vi "Main.vi"() -> ()   [LabVIEW 2017]
uses:
  <vilib>/Platform/TimedLoop/XDataNode/timing_clust.ctl
  <vilib>/Platform/TimedLoop/XDataNode/nitl_modes.ctl
  <vilib>/Platform/TimedLoop/XDataNode/wakeup.ctl
  <instrlib>/_niInstr/Instruction Framework/v1/FPGA/Helper Classes/Single Address Space Collection/Single Address Space Collection.lvclass
  C:/Program Files (x86)/National Instruments/LabVIEW 2017/instr.lib/_niInstr/Instruction Framework/v1/FPGA/Interfaces/Address Space Collection/Address Space Collection.lvclass
  <instrlib>/_niInstr/FIFO Register Bus/v1/FPGA/niInstr FIFO Register Bus v1 FPGA.lvclass
  C:/Program Files (x86)/National Instruments/LabVIEW 2017/instr.lib/_niInstr/Instruction Framework/v1/FPGA/Interfaces/Instruction Producer/Instruction Producer.lvclass
  <vilib>/rvi/Emulation/niFpgaGetClockAttributes.vi
  <vilib>/rvi/Emulation/niFpgaSctlEmulationGetInTimedLoop.vi
  <vilib>/rvi/Emulation/niFpgaEmulationReportErrorSimple.vi
  <vilib>/rvi/eio/common/nirviEmuTemplateMethod_errors.vi
  <vilib>/rvi/Emulation/niFpgaCriticalErrorInLSC.vi
  <vilib>/eio/EIONode/EIONode.xnode
  <vilib>/Platform/TimedLoop/XDataNode/XDataNode.xnode
  <instrlib>/_niInstr/Instruction Framework/v1/FPGA/Top Level Bus/Register Configuration/Register Configuration.lvclass
  Oscillator/Oscillator.lvclass
  <vilib>/Platform/TimedLoop/XDataNode/XDNodeRunTimeDep.lvlib
panel:
  in  "Enable?":bool
  out "Loop":i32
  in  "Signal Offset":i16
  in  "Signal Amplitude (x 2^15)":u16
  in  "Phase Shift":u32
  in  "Accumulator Increment":u32
  in  "Reset Accumulator":bool
  in  "Count(Ticks)":u32
  out "Actual Rate (ticks)":u32
  out "fifo reg bus data 0":u64
  out "fifo reg bus status 0":u32
  in  "fifo reg bus ctrl 0":u32
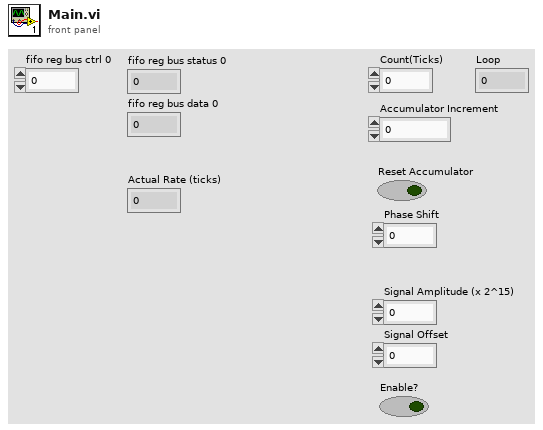
[diagram p1: front panel]
types:
  T1 = typedef "XDNodeRunTimeDep.lvlib/timing_clust.ctl" = cluster{"Expected End [f-1]":u64, "Actual End [f-1]":u64, "Finished Late? [f-1]":bool, "Expected End [i-1]":u64, "Actual End [i-1]":u64, "Finished Late? [i-1]":bool, "Expected Start [i]":u64, "Actual Start [i]":u64, "Expected Start [f]":u64, "Actual Start [f]":u64, "Source Name":string, "Structure Name":string, "Period":i64, "Deadline":i64, "Offset":i64, "Start":i64, "Priority":i32, "Timeout":i32, "Mode":T2, "Wakeup Reason":T3, "Error":errorcluster, "Source Type":string, "Secondary Source Type":string, "Global End Time":u64, "Global Start Time":u64, "Frame Duration":u64, "Iteration Duration":u64, "Assigned CPU":i32, "I/O Scan Engine Mode":u32}
  T2 = typedef "XDNodeRunTimeDep.lvlib/nitl_modes.ctl" = enum32{"No Change", "Process missed periods, maintain original phase", "Discard missed periods, maintain original phase", "Process missed periods, ignore original phase", "Discard missed periods, ignore original phase"}
  T3 = typedef "XDNodeRunTimeDep.lvlib/wakeup.ctl" = enum32{"Normal", "Aborted", "Asynchronous wakeup", "Timing source error", "Timed loop error", "Timeout"}
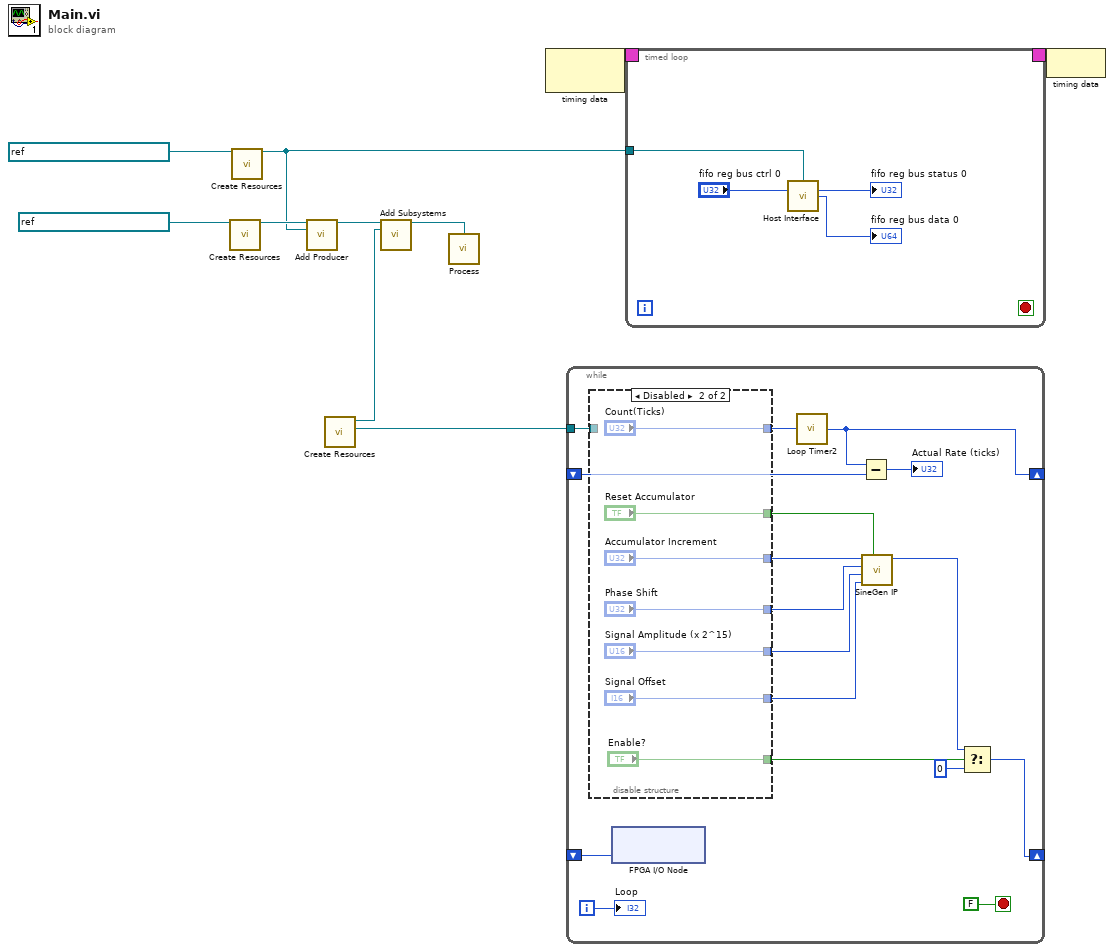
[diagram p0: block diagram]
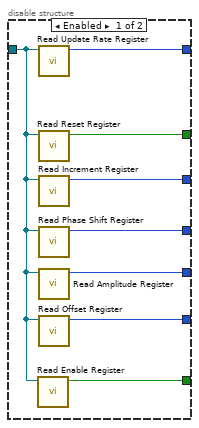
[diagram p2: hidden frame]
diagram:
  n1 = call <instrlib>:"Create Resources.vi"("register clock"=refnum<k21> "40 MHz Onboard Clock") -> ("register configuration"=w7:refnum<class "Register Configuration.lvclass">)  [unwired: 14 in]
  n2 = call <instrlib>:"Create Resources.vi"("instruction fifo"=refnum<k21> "reg.host instruction fifo 0") -> ("fifo register bus"=w5:refnum<class "niInstr FIFO Register Bus v1 FPGA.lvclass">)  [unwired: 14 in]
  n3 = call <instrlib>:"Add Producer.vi"("register configuration in"=w7, "instruction producer"=w5) -> ("register configuration out"=w4:refnum<class "Register Configuration.lvclass">)  [unwired: 13 in]
  n4 = call <instrlib>:"Create Resources.vi"() -> ("Oscillator Address Space out"=w1:refnum<class "Oscillator.lvclass">, "Subsystem out"=w3:refnum<class "Single Address Space Collection.lvclass">)  [unwired: 10 in]
  n5 = call <instrlib>:"Add Subsystems.vi"("register configuration in"=w4, "subsystems"=w3) -> ("register configuration out"=w2:refnum<class "Register Configuration.lvclass">)  [unwired: 13 in]
  n6 = call <instrlib>:"Process.vi"("register configuration"=w2) -> ()  [unwired: 15 in]
  n7 = node-c288() -> (w9:T1)  [unwired: 1 in]
  n8 = while {
    shift-right: [w12] -> _
    shift-left: _ -> [w27]
    shift-right: [w25] -> _
    shift-left: _ -> [w26]
    tunnel: w1 -> [w17]
    i -> [w15]
    stop <- FALSE stop-if-true
    n9 = disable-structure shown="Disabled" {
      disable-tunnel: [w35 "Count(Ticks)"] -> w22
      disable-tunnel: [w34 "Signal Amplitude (x 2^15)"] -> w21
      disable-tunnel: [w33 "Phase Shift"] -> w20
      disable-tunnel: [w32 "Accumulator Increment"] -> w19
      disable-tunnel: [w31 "Reset Accumulator"] -> w18
      disable-tunnel: w17 -> [w29 _]
      disable-tunnel: [w30 "Signal Offset"] -> w16
      disable-tunnel: [w28 "Enable?"] -> w14
      frame Enabled {
        n10 = call "Read Enable Register.vi"("Oscillator Address Space in"=w29) -> ("reset"=w28:bool)  [unwired: 10 in]
        n11 = call "Read Update Rate Register.vi"("Oscillator Address Space in"=w29) -> ("phase shift"=w35:u32)  [unwired: 10 in]
        n12 = call "Read Reset Register.vi"("Oscillator Address Space in"=w29) -> ("reset"=w31:bool)  [unwired: 10 in]
        n13 = call "Read Increment Register.vi"("Oscillator Address Space in"=w29) -> ("increment"=w32:u32)  [unwired: 10 in]
        n14 = call "Read Phase Shift Register.vi"("Oscillator Address Space in"=w29) -> ("phase shift"=w33:u32)  [unwired: 10 in]
        n15 = call "Read Amplitude Register.vi"("Oscillator Address Space in"=w29) -> ("amplitude"=w34:u16)  [unwired: 10 in]
        n16 = call "Read Offset Register.vi"("Oscillator Address Space in"=w29) -> ("amplitude"=w30:i16)  [unwired: 10 in]
      }
      frame Disabled {
      }
    }
    n17 = xnode "FPGA I/O Node"("Oscillator"=w27) -> ()  [unwired: 1 in, 1 out]
    n18 = call "Loop Timer2"("Count(Ticks)"=w22) -> ("Tick Count(Ticks)"=w25:u32)
    n19 = Subtract(x=w25, y=w26) -> (x-y=→"Actual Rate (ticks)":u32)
    n20 = call "SineGen IP.vi"("Reset Accumulator"=w18, "Signal Offset"=w16, "Signal Amplitude (x 2^15)"=w21, "Phase Shift"=w20, "Accumulator Increment"=w19) -> ("Signal Value"=w13:i16)  [unwired: 5 in, 1 out]
    n21 = Select(t=w13, s=w14, f=i16 0) -> (s? t:f=w12:i16)
    "Loop" <- w15
  }
  n22 = timed-loop {
    timing: w9 -> [_]
    timing-out: [_] -> w8
    tunnel: w5 -> [w46]
    stop <- _ stop-if-true
    n23 = call <instrlib>:"Host Interface.vi"("fifo register bus"=w46, "fifo reg bus ctrl 0"="fifo reg bus ctrl 0") -> ("fifo reg bus status 0"=→"fifo reg bus status 0":u32, "fifo reg bus data 0"=→"fifo reg bus data 0":u64)  [unwired: 12 in]
  }
  n24 = node-c288(w8) -> ()
